vi "Write Broadcast Period.vi"(8 "error in (no error)":errorcluster, 10 "Broadcast Period":u32, 11 "Device Connector in":refnum<class "Device Connector.lvclass">) -> (0 "error out":errorcluster, 3 "Device Connector out":refnum<class "Device Connector.lvclass">)   [LabVIEW 2024, in "Device Connector.lvclass"]
uses:
  Device Connector.lvclass
  Device Connector.lvclass/Device Connector.ctl
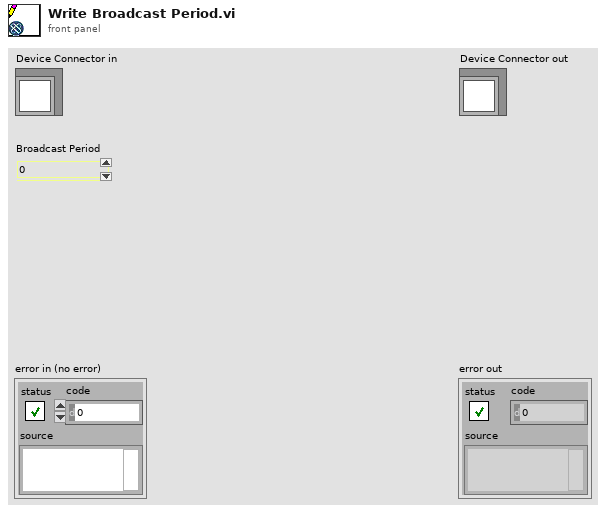
[diagram p1: front panel]
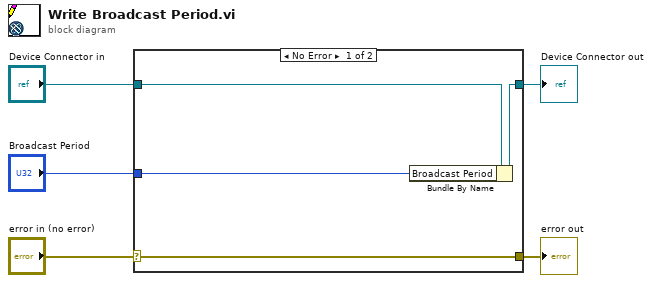
[diagram p0: block diagram]
diagram:
  n1 = case shown="No Error" "error in (no error)" {
    selector: "error in (no error)" -> [w9 w10]
    tunnel: [w9 w10] -> w4
    tunnel: [w7 w11] -> w2
    tunnel: "Device Connector in" -> [w8 w11]
    tunnel: "Broadcast Period" -> [w6 _]
    frame No Error {
      n2 = Bundle By Name(cluster=w8, "Broadcast Period"=w6) -> (w7:refnum<class "Device Connector.lvclass">)
    }
    frame Error {
    }
  }
  "error out" <- w4
  "Device Connector out" <- w2
